vi "RageAte_Delay_w-ProgressBar-2.vi"(6 "Seconds":i32, 8 "error in (no error)":errorcluster, 10 "Delay text ...":string="Temperature soaking...") -> (0 "error out":errorcluster)   [LabVIEW 2018]
uses:
  System.Windows.Forms
panel:
  in  "Skip":bool
  in  "Step":i32=25
  out "Caption":refnum<vi>
  in  "ProgressBar":refnum<k24>(container)
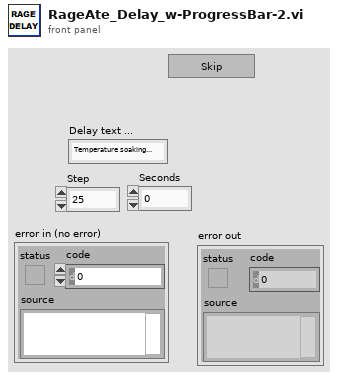
[diagram p1: front panel]
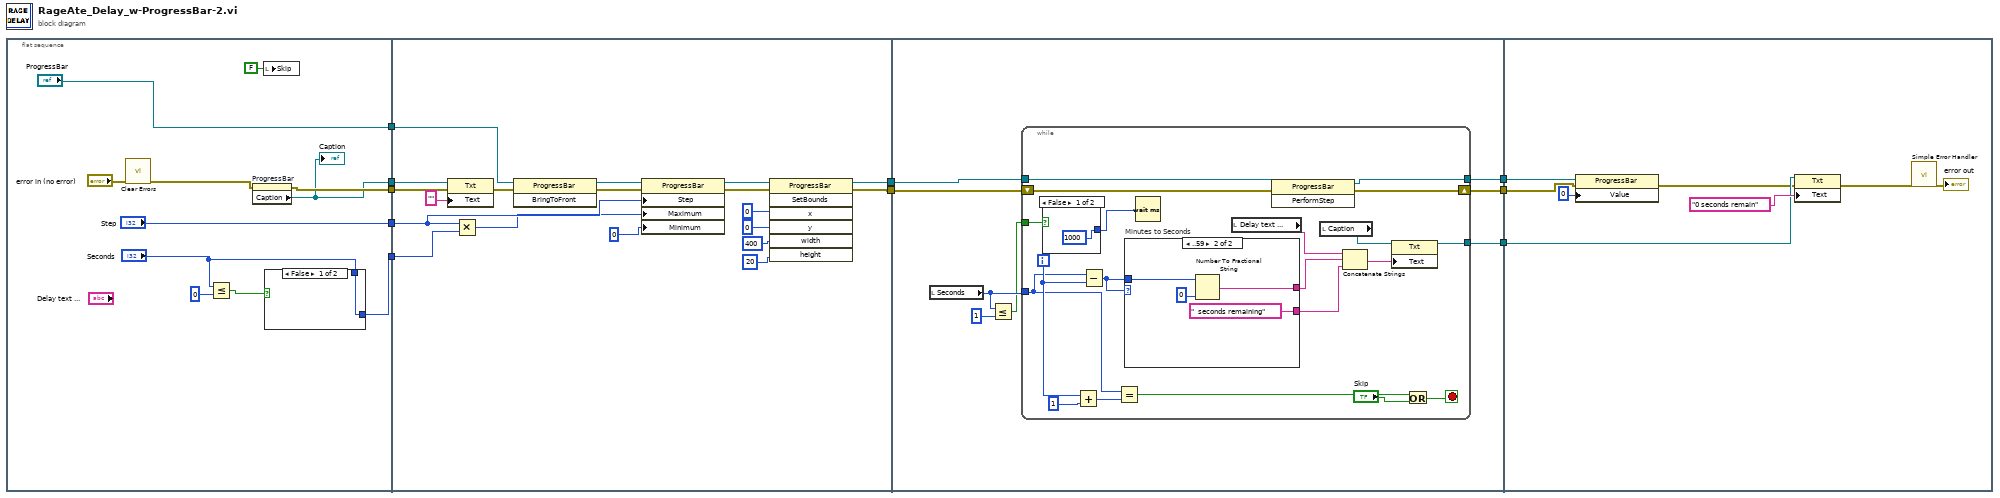
[diagram p0: block diagram]
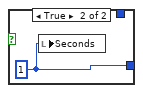
[diagram p2: hidden frame]
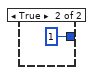
[diagram p3: hidden frame]
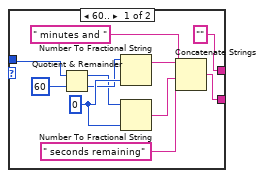
[diagram p4: hidden frame]
diagram:
  n1 = flat-sequence {
    tunnel: [w14] -> w5
    tunnel: ["Step"] -> w4
    tunnel: [w20] -> w3
    tunnel: [w19] -> w2
    tunnel: ["ProgressBar"] -> w1
    tunnel: [w38] -> w10
    tunnel: [w34] -> w9
    tunnel: w5 -> [w31]
    tunnel: w4 -> [w25]
    tunnel: w3 -> [w30]
    tunnel: w2 -> [w33]
    tunnel: w1 -> [w26]
    tunnel: w10 -> [w49]
    tunnel: w9 -> [w50]
    tunnel: [w48] -> w8
    tunnel: [w47] -> w7
    tunnel: [w46] -> w6
    tunnel: w8 -> [w93]
    tunnel: w7 -> [w92]
    tunnel: w6 -> [w91]
    frame #0 {
      n2 = call <vilib>:"Clear Errors.vi"("error in (no error)"="error in (no error)") -> ("error out"=w16:errorcluster)  [unwired: 5 in, 1 out]
      n3 = Less Or Equal?(x="Seconds", y=0) -> (x <= y?=w12:bool)
      n4 = property on="ProgressBar" class="AXCont"(error in=w16) -> (error out=w20:errorcluster, "Caption"=w19:refnum<vi>)  [unwired: 1 in, 1 out]
      "Caption" <- w19
      n5 = local write "Skip"(FALSE ("stop")) -> ()
      n6 = case shown="False" w12 {
        tunnel: [w22 w23] -> w14
        tunnel: "Seconds" -> [w22 _]
        frame False {
        }
        frame True {
          w23 = 1
          n7 = local write "Seconds"(w23) -> ()
        }
      }
    }
    frame #1 {
      n8 = property class="Txt"(reference=w33, error in=w30, "Text"="") -> (error out=w28:errorcluster)  [unwired: 1 out]
      n9 = Multiply(x=w25, y=w31) -> (x*y=w24:i32)
      n10 = invoke class="ProgressBar" method="BringToFront"(reference=w26, error in=w28) -> (reference out=w29:refnum<k24>, error out=w27:errorcluster)  [unwired: 1 in, 1 out]
      n11 = property class="ProgressBar"(reference=w29, error in=w27, "Step"=w25, "Maximum"=w24, "Minimum"=0) -> (reference out=w36:refnum<k24>, error out=w35:errorcluster)
      n12 = invoke class="ProgressBar" method="SetBounds"(reference=w36, error in=w35, "x"=0, "y"=0, "width"=400, "height"=20) -> (reference out=w38:refnum<k24>, error out=w34:errorcluster)  [unwired: 1 in, 5 out]
    }
    frame #2 {
      n13 = local read "Seconds"() -> (w45:i32)
      n14 = Less Or Equal?(x=w45, y=1) -> (x <= y?=w43:bool)
      n15 = while {
        tunnel: w49 -> [w67]
        shift-right: [w62] -> w47
        shift-left: w50 -> [w70]
        tunnel: [w68] -> w48
        tunnel: [w61] -> w46
        tunnel: w45 -> [w55]
        tunnel: w43 -> [w51]
        i -> [w60]
        stop <- w58 stop-if-true
        n16 = case shown="False" w51 {
          tunnel: [u32 1000 ("milliseconds to wait") u32 1 ("milliseconds to wait")] -> w69
          frame False {
          }
          frame True {
          }
        }
        n17 = Add(x=w60, y=1) -> (x+y=w54:i32)
        n18 = Subtract(x=w55, y=w60) -> (x-y=w53:i32)
        n19 = Equal?(x=w55, y=w54) -> (x = y?=w59:bool)
        n20 = case "Minutes to Seconds" shown="..59" w53 {
          tunnel: w53 -> [w76 w87]
          tunnel: ["" w86] -> w66
          tunnel: [w78 "  seconds remaining" ("string")] -> w65
          frame 60.. {
            w83 = i16 0 ("precision (6)")
            n21 = Quotient & Remainder(x=w76, y=60) -> (x-y*floor(x/y)=w73:i32, floor(x/y)=w74:i32)
            n22 = Number To Fractional String(number=w74, precision (6)=w83) -> (F-format string=w79:string)  [unwired: 2 in]
            n23 = Number To Fractional String(number=w73, precision (6)=w83) -> (F-format string=w81:string)  [unwired: 2 in]
            n24 = Concatenate Strings(w79, " minutes and " ("string"), w81, " seconds remaining" ("string")) -> (w78:string)
          }
          frame ..59 {
            n25 = Number To Fractional String(number=w87, precision (6)=i16 0) -> (F-format string=w86:string)  [unwired: 2 in]
          }
        }
        n26 = Wait (ms)(milliseconds to wait=w69) -> ()  [unwired: 1 out]
        n27 = local read "Delay text ..."() -> (w52:string)
        n28 = invoke class="ProgressBar" method="PerformStep"(reference=w67, error in=w70) -> (reference out=w68:refnum<k24>, error out=w62:errorcluster)  [unwired: 1 in, 1 out]
        n29 = local read "Caption"() -> (w63:refnum<vi>)
        n30 = Concatenate Strings(w52, w66, w65) -> (w64:string)
        n31 = property class="Txt"(reference=w63, "Text"=w64) -> (reference out=w61:refnum<vi>)  [unwired: 1 in, 1 out]
        n32 = Or(x=w59, y="Skip") -> (x .or. y?=w58:bool)
      }
    }
    frame #3 {
      n33 = property class="ProgressBar"(reference=w93, error in=w92, "Value"=0) -> (error out=w89:errorcluster)  [unwired: 1 out]
      n34 = property class="Txt"(reference=w91, error in=w89, "Text"="0 seconds remain") -> (error out=w88:errorcluster)  [unwired: 1 out]
      n35 = call <vilib>:"Simple Error Handler.vi"("error in (no error)"=w88) -> ("error out"=→"error out":errorcluster)  [unwired: 4 in, 4 out]
    }
  }
